vi "tearDown.vi"(8 "error in (no error)":errorcluster, 11 "reference in":refnum<class "TestSQliteDatabaseConfiguration.lvclass">) -> (0 "error out":errorcluster, 3 "reference out":refnum<class "TestSQliteDatabaseConfiguration.lvclass">)   [LabVIEW 2020, in "SQlite tests.lvlib" / "TestSQliteDatabaseConfiguration.lvclass"]
doc: "tearDown runs after the test method has completed. Use this method to clean up any operations or references that were opened by setUp or the test method. Unit tests should be independent of other unit tests so this VI should ensure that the next test can run in a 'clean' test environment."
uses:
  TestSQliteDatabaseConfiguration.lvclass
  TestSQliteDatabaseConfiguration.lvclass/TestSQliteDatabaseConfiguration.ctl
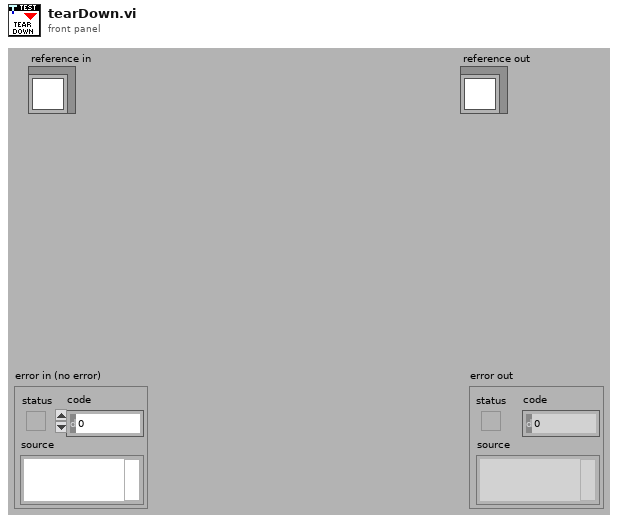
[diagram p1: front panel]
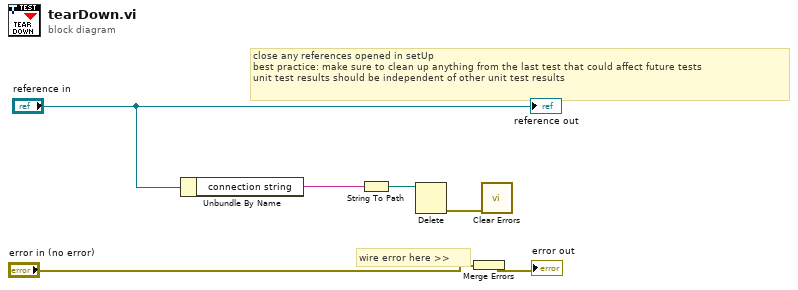
[diagram p0: block diagram]
diagram:
  # "wire error here >>"
  # "close any references opened in setUp\nbest practice: make sure to clean up anything from the last test that could affect future tests\nunit test results should be independent of other unit test results"
  n1 = Unbundle By Name("reference in") -> ("connection string"=w2:string)
  n2 = String To Path(string=w2) -> (path=w1:path)
  n3 = Delete(path (use dialog)=w1) -> (error out=w3:errorcluster)  [unwired: 4 in, 2 out]
  n4 = Merge Errors("error in (no error)") -> (→"error out":errorcluster)
  n5 = call <vilib>:"Clear Errors.vi"("error in (no error)"=w3) -> ()  [unwired: 5 in, 2 out]
  "reference out" <- "reference in"
